vi "RC Decay acquisition loop.vi"(7 "Timing Control Parameters In":T1={"N cycles for averaging"=100, "N points per measurement"=1000, "Measurment time interval"=1e-05} {"Measurment time interval" format="%.2e"}, 11 "error in (no error)":errorcluster) -> (3 "time-out?":bool, 4 "data valid":bool=TRUE, 8 "Normalized Waveform Out":waveform(dbl)={"t0"=timestamp(3255113673.8489995 s since 1904-01-01), "dt"=9.999999747378752e-06, "Y"=array[1000 elements]}, 10 "Timing Control Parameters Out":T1={"N cycles for averaging"=300, "N points per measurement"=1000, "Measurment time interval"=1e-05} {"Measurment time interval" format="%.2e"}, 15 "error out":errorcluster)   [LabVIEW 2016]
doc: "This subvi manages the capacitance measurement\n\nPaul K Dixon\nPhysics 350\nCSUSB Physics"
uses:
  globals/C(T) global variables.vi
panel:
  out "data":waveform(dbl)[](array[waveform])=[{"t0"=timestamp(3255113673.8489995 s since 1904-01-01), "dt"=9.999999747378752e-06, "Y"=array[1000 elements], "attributes"=variant("NI_ChannelName"=variant(string "1"), "NI_DeviceNumber"=variant(i32 1), "NI_UnitDescription"=variant(string "Volts"))}, {"t0"=timestamp(3255113673.8489995 s since 1904-01-01), "dt"=9.999999747378752e-06, "Y"=array[1000 elements], "attributes"=variant("NI_ChannelName"=variant(string "2"), "NI_DeviceNumber"=variant(i32 1), "NI_UnitDescription"=variant(string "Volts"))}] caption="Individual Waveforms"
  out "Individual Waveforms":waveform(dbl)[](graph)
  out "Final Waveform":waveform(dbl)(graph)={"t0"=timestamp(3255113673.8489995 s since 1904-01-01), "dt"=9.999999747378752e-06, "Y"=[]}
  out "loop index":i32=300
  out "scan rate (Hz)":dbl=99999.99999999999 format="%.2e"
  out "meas index":i32=300
  in  "Proceed":bool
  # "RC Decay Acquisition for C(T) Experiment"
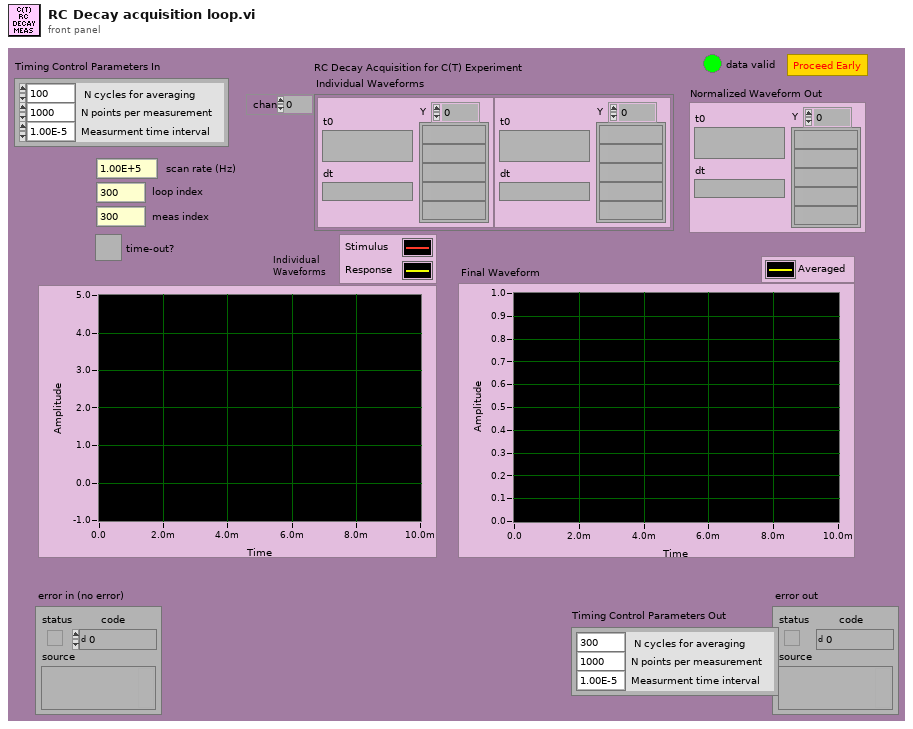
[diagram p1: front panel]
types:
  T1 = cluster{"N cycles for averaging":i32, "N points per measurement":i32, "Measurment time interval":dbl}
  T2 = enum16{"AI sample channel scan", "AI Waveform triggered"}
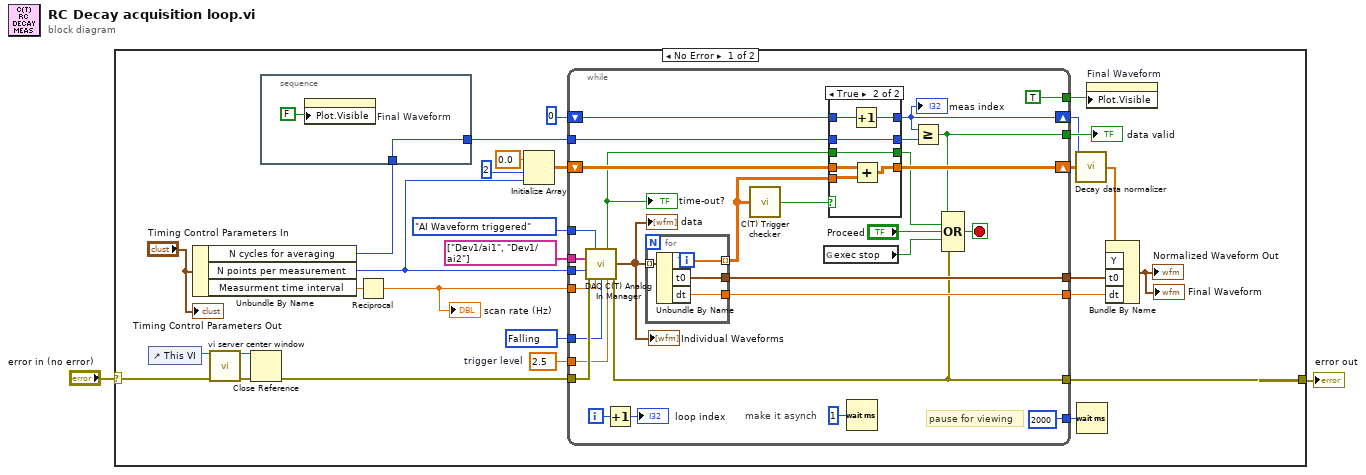
[diagram p0: block diagram]
diagram:
  n1 = case shown="No Error" "error in (no error)" {
    selector: "error in (no error)" -> [w8 w79]
    tunnel: [w5 w79] -> w2
    frame No Error {
      w13 = 2.5  # trigger level
      w9 = 10171 items=["Rising"=10280, "Falling"=10171] ("trigger edge")
      n2 = control-ref of="This VI"() -> (w7:refnum<vi>)
      n3 = Unbundle By Name("Timing Control Parameters In") -> ("N cycles for averaging"=w16:i32, "N points per measurement"=w23:i32, "Measurment time interval"=w25:dbl)
      n4 = call "vi server center window.vi"("VI ref in"=w7, "error in"=w8) -> ("VI ref out"=w3:refnum<vi>, "error out"=w6:errorcluster)  [unwired: 12 out]
      n5 = Close Reference(reference=w3, error in (no error)=w6) -> (error out=w4:errorcluster)
      n6 = stacked-sequence {
        tunnel: [w77] -> w15
        tunnel: w16 -> [w77]
        frame #0 {
          n7 = property on="Final Waveform" class="WFGraph (strict)"("Plot.Visible"=FALSE) -> ()  [unwired: 2 in, 2 out]
        }
      }
      n8 = Reciprocal(x=w25) -> (1/x=w24:dbl)
      "scan rate (Hz)" <- w24
      n9 = Initialize Array(0.0 ("Element Data"), 2 ("Dimension Size"), w23) -> (w29:dbl[][])
      n10 = while {
        tunnel: [TRUE ("Plot.Visible")] -> w14
        tunnel: [w46] -> w17
        tunnel: [w47] -> w12
        tunnel: [w49] -> w22
        tunnel: w15 -> [w53]
        shift-left: 0 ("Dimension Size") -> [w56]
        shift-right: [w52] -> w20
        tunnel: w24 -> [w58]
        tunnel: T2."AI Waveform triggered" ("AI mode chooser") -> [w59]
        tunnel: w23 -> [w60]
        shift-left: w29 -> [w55]
        shift-right: [w54] -> w21
        tunnel: w13 -> [w41]
        tunnel: [u32 2000 ("milliseconds to wait")] -> w11
        tunnel: w4 -> [w61]
        tunnel: [w32] -> w5
        tunnel: tag[] ["Dev1/ai1", "Dev1/ai2"] ("Channels (Triggered Waveform)") -> [w34]
        tunnel: w9 -> [w33]
        i -> [w50]
        stop <- w38 stop-if-true
        # "pause for viewing"
        # "make it asynch"
        n11 = call "DAQ C(T) Analog In Manager.vi"("AI mode chooser"=w59, "Channels (Triggered Waveform)"=w34, "number of scans to acquire"=w60, "error in (no error)"=w61, "scan rate"=w58, "trigger edge"=w33, "trigger level"=w41) -> ("Timed Out"=w35:bool, "data"=w43:waveform(dbl)[], "error out"=w32:errorcluster)  [unwired: 4 in, 2 out]
        "time-out?" <- w35
        "Individual Waveforms" <- w43
        "data" <- w43
        n12 = Increment(x=w50) -> (x+1=→"loop index":i32)
        n13 = for {
          tunnel: w43 -> [w76] mode=indexing
          tunnel: [w73] -> w40 mode=indexing
          tunnel: [w74] -> w47
          tunnel: [w75] -> w46
          n14 = Unbundle By Name(w76) -> ("Y"=w73:dbl[], "t0"=w74:timestamp, "dt"=w75:dbl)
        }
        n15 = call "C(T) Trigger checker.vi"("Raw C(T) data array"=w40) -> ("trigger was correct polarity"=w57:bool)
        n16 = global read "C(T) global variables.vi" "exec stop"() -> (w37:bool)
        n17 = case shown="True" w57 {
          tunnel: w40 -> [_ w69]
          tunnel: w56 -> [w65 w72]
          tunnel: [w65 w71] -> w52
          tunnel: w55 -> [w64 w70]
          tunnel: [w64 w68] -> w54
          tunnel: [w63 w67] -> w51
          tunnel: w53 -> [w63 w67]
          tunnel: [w62 w66] -> w36
          tunnel: w35 -> [w62 w66]
          frame False {
          }
          frame True {
            n18 = Increment(x=w72) -> (x+1=w71:i32)
            n19 = Add(x=w70, y=w69) -> (x+y=w68:dbl[][])
          }
        }
        "meas index" <- w52
        n20 = Wait (ms)(milliseconds to wait=u32 1) -> ()  [unwired: 1 out]
        n21 = Greater Or Equal?(x=w52, y=w51) -> (x >= y?=w49:bool)
        n22 = Compound Arithmetic op=OR(w49, w36, "Proceed", w37, w32) -> (w38:bool)
      }
      "data valid" <- w22
      n23 = call "Decay data normalizer.vi"("Number of samples"=w20, "Raw summed data Array"=w21) -> ("Normalized Decay"=w18:dbl[])  [unwired: 13 out]
      n24 = Wait (ms)(milliseconds to wait=w11) -> ()  [unwired: 1 out]
      n25 = property on="Final Waveform" class="WFGraph (strict)"("Plot.Visible"=w14) -> ()  [unwired: 2 in, 2 out]
      n26 = Bundle By Name("Y"=w18, "t0"=w12, "dt"=w17) -> (→"Normalized Waveform Out" →"Final Waveform":waveform(dbl))  [unwired: 1 out]
      "Timing Control Parameters Out" <- "Timing Control Parameters In"
    }
    frame Error {
    }
  }
  "error out" <- w2
